vi "ObtainRequestEvents.vi"(8 "error in (no error)":errorcluster) -> (0 "error out":errorcluster, 2 "clRequestEvents":T1)   [LabVIEW 2014, in "PmuImpairModule.lvlib"]
uses:
  PmuImpairModule.lvlib
  clRequestEvents.ctl
  clEventType.ctl
panel:
  # "If you want to add other Request Events, open this typedef, copy an existing event and rename it to your Request name.\n\nNext create a typedef for the  data and put it into PublicAPI/Arguments/Requests\n\nNext, add an event handler loop event case in Main.vi to handle the new request event\n\nMost likely, each request will also require the creation of a new Queued Message Handler loop case in Main.VI"
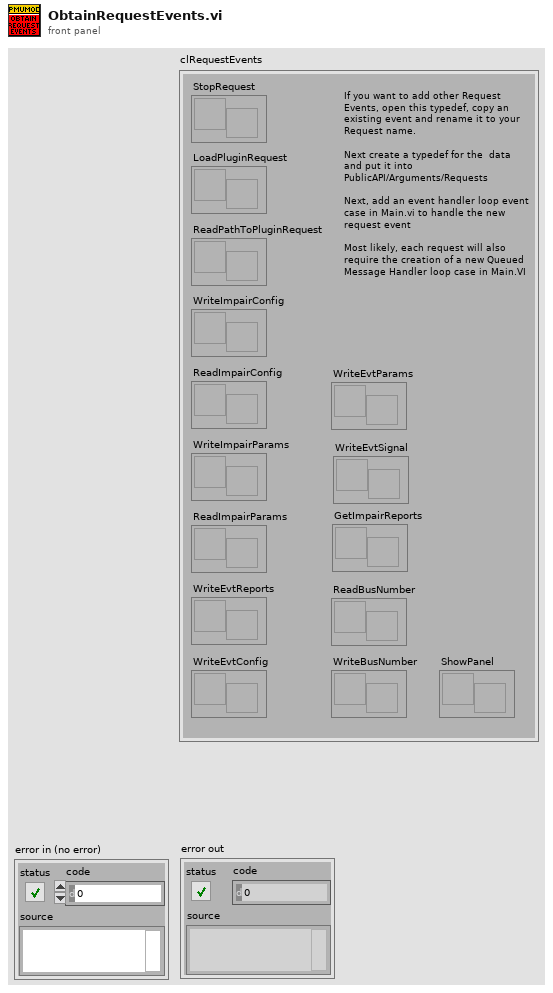
[diagram p1: front panel]
types:
  T1 = typedef "PmuImpairModule.lvlib/clRequestEvents.ctl" = cluster{"StopRequest":refnum<user-event>, "LoadPluginRequest":refnum<user-event>, "WriteImpairConfig":refnum<user-event>, "ReadImpairConfig":refnum<user-event>, "WriteImpairParams":refnum<user-event>, "ReadImpairParams":refnum<user-event>, "WriteEvtReports":refnum<user-event>, "GetImpairReports":refnum<user-event>, "ReadPathToPluginRequest":refnum<user-event>, "WriteEvtSignal":refnum<user-event>, "WriteEvtConfig":refnum<user-event>, "WriteEvtParams":refnum<user-event>, "ReadBusNumber":refnum<user-event>, "WriteBusNumber":refnum<user-event>, "ShowPanel":refnum<user-event>}
  T2 = typedef "PmuImpairModule.lvlib/clEventType.ctl" = cluster{"ModuleID":i32, "Data":variant}
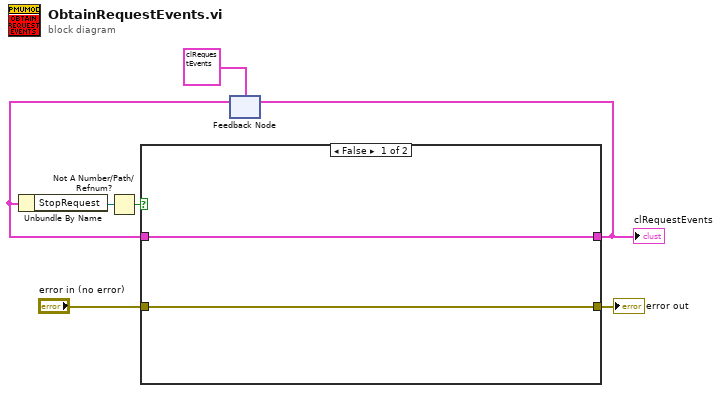
[diagram p0: block diagram]
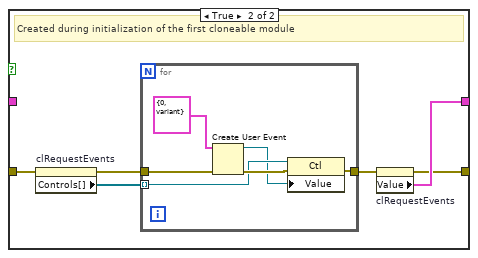
[diagram p2: hidden frame]
diagram:
  n1 = feedback #1(T1 {"StopRequest"=refnum, "LoadPluginRequest"=refnum, "WriteImpairConfig"=refnum, "ReadImpairConfig"=refnum, "WriteImpairParams"=refnum, "ReadImpairParams"=refnum, "WriteEvtReports"=refnum, "GetImpairReports"=refnum, "ReadPathToPluginRequest"=refnum, "WriteEvtSignal"=refnum, "WriteEvtConfig"=refnum, "WriteEvtParams"=refnum, "ReadBusNumber"=refnum, "WriteBusNumber"=refnum, "ShowPanel"=refnum} ("Value")) -> (w4:T1)
  n2 = Unbundle By Name(w4) -> ("StopRequest"=w1:refnum<user-event>)
  n3 = Not A Number/Path/Refnum?(number/path/refnum=w1) -> (NaN/Path/Refnum?=w2:bool)
  n4 = case shown="False" w2 {
    tunnel: "error in (no error)" -> [w9 w15]
    tunnel: w4 -> [w8 _]
    tunnel: [w9 w10] -> w6
    tunnel: [w8 w12] -> w5
    frame False {
    }
    frame True {
      # "Created during initialization of the first cloneable module"
      n5 = property on="clRequestEvents" class="Clust (strict)"(error in=w15) -> (error out=w13:errorcluster, "Controls[]"=w14:refnum<vi>[])  [unwired: 1 in, 1 out]
      n6 = for {
        tunnel: w14 -> [w17] mode=indexing
        tunnel: w13 -> [w20]
        tunnel: [w18] -> w11
        n7 = Create User Event(user event datatype=T2 {"ModuleID"=0, "Data"=variant} ("clEventType"), error in=w20) -> (user event=w16:refnum<user-event>, error out=w19:errorcluster)
        n8 = property on="Property Node" class="Ctl"(reference=w17, error in=w19, "Value"=w16) -> (error out=w18:errorcluster)  [unwired: 1 out]
      }
      n9 = property on="clRequestEvents" class="Clust (strict)"(error in=w11) -> (error out=w10:errorcluster, "Value"=w12:T1)  [unwired: 1 in, 1 out]
    }
  }
  "error out" <- w6
  "clRequestEvents" <- w5
  n10 = feedback-in #1(w5) -> ()
